vi "EQE_Scan.vi"(4 "Max loop":i32=20, 5 "error in (no error)":errorcluster, 6 "milliseconds to wait":u32=150, 7 "Long delay":bool, 8 "Wavelength":dbl=300.0, 9 "VISA Lock-in":refnum<visa-resource-name>) -> (0 "error out":errorcluster, 1 "Error Code":i32, 2 "Output bundle":cluster{"Wavelength":dbl, "R":dbl})   [LabVIEW 2017]
panel:
  out "Lock-in Value":dbl
  out "Current Wavelength":dbl
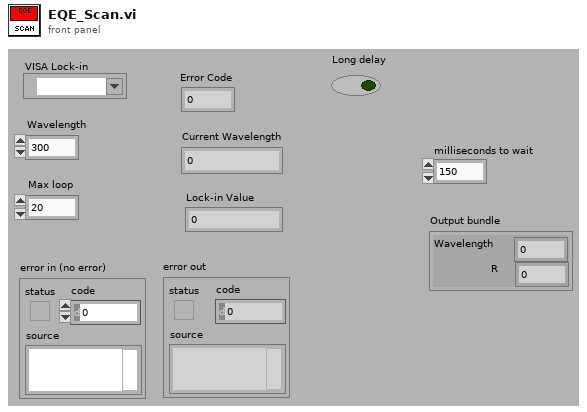
[diagram p1: front panel]
types:
  T1 = cluster{"Current Wavelength":dbl, "1 parameter (final mean)":dbl}
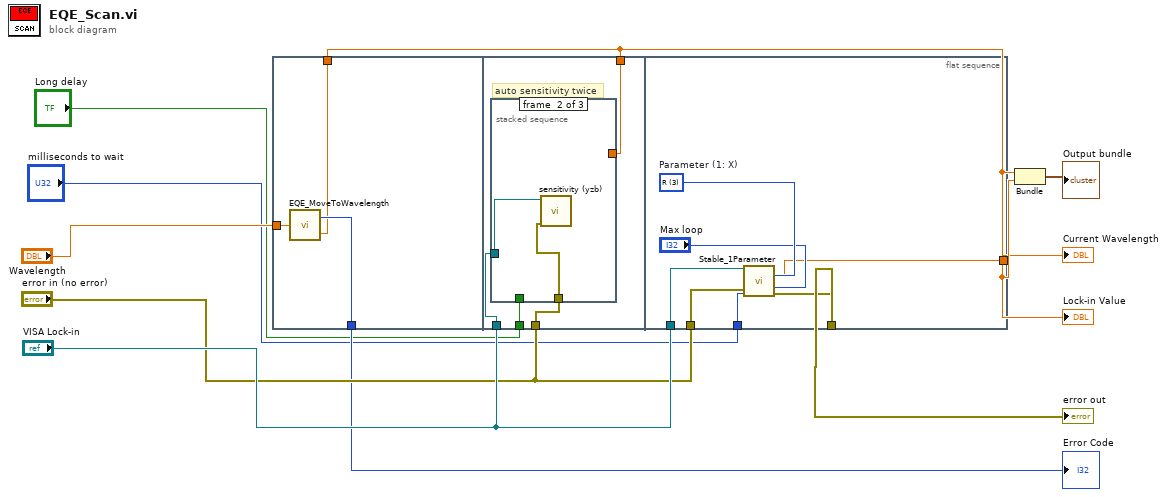
[diagram p0: block diagram]
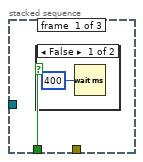
[diagram p2: hidden frame]
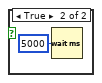
[diagram p3: hidden frame]
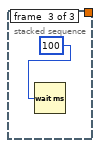
[diagram p4: hidden frame]
diagram:
  n1 = flat-sequence {
    tunnel: [w13] -> w6
    tunnel: "Wavelength" -> [w12]
    tunnel: [w11] -> w3
    tunnel: "VISA Lock-in" -> [w17]
    tunnel: "error in (no error)" -> [w16]
    tunnel: w3 -> [w15]
    tunnel: "Long delay" -> [w14]
    tunnel: "VISA Lock-in" -> [w30]
    tunnel: "error in (no error)" -> [w29]
    tunnel: [w28] -> w10
    tunnel: [w25] -> w5
    tunnel: "milliseconds to wait" -> [w24]
    frame #0 {
      n2 = call "EQE_MoveToWavelength.vi"("Input Wavelength"=w12) -> ("Error Code"=w13:i32, "Current Wavelength"=w11:dbl)
    }
    frame #1 {
      # "auto sensitivity twice"
      n3 = stacked-sequence {
        tunnel: w17 -> [_ w22 _]
        tunnel: w16 -> [_ w21 _]
        tunnel: w15 -> [_ _ _]
        tunnel: w14 -> [w18 _ _]
        frame #0 {
          n4 = case shown="False" w18 {
            frame False {
              n5 = Wait (ms)(milliseconds to wait=u32 400) -> ()  [unwired: 1 out]
            }
            frame True {
              n6 = Wait (ms)(milliseconds to wait=u32 5000) -> ()  [unwired: 1 out]
            }
          }
        }
        frame #1 {
          n7 = call "sensitivity (yzb).vi"("error in (no error)"=w21, "VISA resource name"=w22) -> ()  [unwired: 8 in, 2 out]
        }
        frame #2 {
          n8 = Wait (ms)(milliseconds to wait=u32 100) -> ()  [unwired: 1 out]
        }
      }
    }
    frame #2 {
      w27 = u16 3 items=["X"=1, "Y"=2, "R"=3, "Theta"=4, "Channel 1"=5, "Channel 2"=6, "Aux In 1"=7, "Aux In 2"=8, "Aux In 3"=9, "Aux In 4"=10]  # Parameter (1: X)
      n9 = call "Stable_1Parameter.vi"("VISA resource name"=w30, "Parameter (1: X)"=w27, "Max loop n"="Max loop", "milliseconds to wait"=w24, "error in (no error)"=w29) -> ("1 parameter (final mean)"=w25:dbl, "error out"=w28:errorcluster)  [unwired: 8 in, 1 out]
    }
  }
  n10 = Bundle("Current Wavelength"=w3, "1 parameter (final mean)"=w5) -> (→"Output bundle":T1)  [unwired: 1 in]
  "Error Code" <- w6
  "error out" <- w10
  "Lock-in Value" <- w5
  "Current Wavelength" <- w3
